vi "UpdateClassIcon.vi"() -> ()   [LabVIEW 2020]
uses:
  <resource>/Framework/Providers/API/mxLvChangeType.ctl
panel:
  out "error out":errorcluster
  out "Name":string
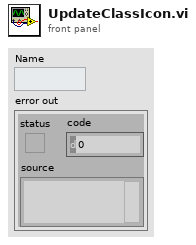
[diagram p1: front panel]
types:
  T1 = typedef "mxLvChangeType.ctl" = enum32{"Item Created", "Item Modified", "File Modified", "File Deleted", "Item Added", "Item Added to SCC", "Item Renamed", "Item Modified For SCC"}
  T2 = cluster{"Item URL":string, "Item ID":string, "Item Index":i32, "Specific Type":string}
  T3 = typedef "ItemRef.ctl" = u64
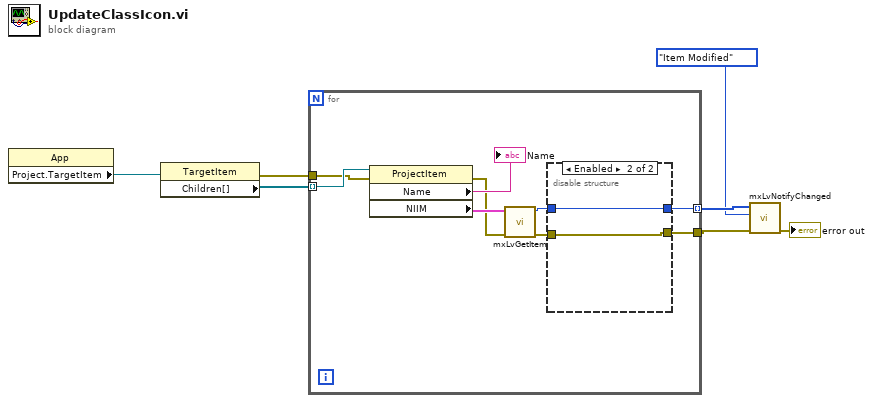
[diagram p0: block diagram]
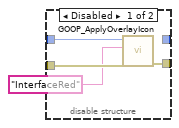
[diagram p2: hidden frame]
diagram:
  n1 = property class="App"() -> ("Project.TargetItem"=w7:refnum<vi>)  [unwired: 2 in, 2 out]
  n2 = property class="TargetItem"(reference=w7) -> (error out=w5:errorcluster, "Children[]"=w6:refnum<vi>[])  [unwired: 1 in, 1 out]
  n3 = for {
    tunnel: w6 -> [w16] mode=indexing
    tunnel: w5 -> [w14]
    tunnel: [w9] -> w3
    tunnel: [w8] -> w4 mode=indexing
    n4 = property class="ProjectItem"(reference=w16, error in=w14) -> (error out=w12:errorcluster, "Name"=→"Name":string, "NIIM"=w15:T2)  [unwired: 1 out]
    n5 = call <resource>:"mxLvGetItem.vi"("error in"=w12, "NIIM"=w15) -> ("error out"=w11:errorcluster, "Item"=w10:T3)  [unwired: 8 in]
    n6 = disable-structure shown="Enabled" {
      disable-tunnel: w11 -> [w20 w22]
      disable-tunnel: w10 -> [w19 w21]
      disable-tunnel: [w18 w22] -> w9
      disable-tunnel: [_ w21] -> w8
      frame Disabled {
        n7 = call <resource>:"GOOP_ApplyOverlayIcon.vi"("error in (no error)"=w20, "IconName(NoPngExtension)"="InterfaceRed", "Object"=w19) -> ("error out"=w18:errorcluster)  [unwired: 8 in]
      }
      frame Enabled {
      }
    }
  }
  n8 = call <resource>:"mxLvNotifyChanged.vi"("error in (no error)"=w3, "Change Type"=mxLvChangeType."Item Modified", "Items"=w4) -> ("error out"=→"error out":errorcluster)  [unwired: 7 in, 1 out]
